vi "fftw__malloc_cplx_poly.vi"   [LabVIEW 2020, in "FFTWDLL.lvlib"]
doc: "Allocate FFTW aligned array of complex reals."
uses:
  FFTWDLL.lvlib
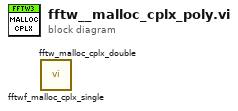
[diagram p0: block diagram]
diagram:
  n1 = call "fftwf_malloc_cplx_single.vi"() -> ()  [unwired: 10 in, 2 out]
  n2 = call "fftw_malloc_cplx_double.vi"() -> ()  [unwired: 10 in, 2 out]
